vi "File Manager.vi"(0 "File Name":string, 1 "File Choice":T3, 3 "Existing Time":dbl, 4 "Voltage":waveform(dbl)[](array[waveform]), 5 "error in":errorcluster, 6 "Enum":T2=enum."Close File", 7 "Record Time (s)":dbl=10.0, 12 "Volt Channel":T1={"Index"=[], "Chl Name"=[], "Scale"=[], "Offset"=[], "Sample Rate"=100, "Device Name"="", "Channel"=""}, 13 "Use Record Time":bool) -> (14 "File Path":path, 15 "timeout":i32, 16 "ET out":dbl, 17 "Recording":bool, 18 "dt Out":dbl, 19 "error out":errorcluster)   [LabVIEW 2021]
doc: "This vi has four functions:\nCreate File - Create a new TDMS or CSV file depending on user choice. If user filled in file name, use that file name with time infomation. If user didn't filled in file name, use \"Experiment Result \"+time information.\nConfig Data - Save Channel Number, Channel Name, Scale and Offset into file.\nVolt Data - Create Time array and merge with Voltage Data, then save them into file. \nClost File - Close file and reset all parameters."
uses:
  Control/File Choice Enum.ctl
  Control/File Manager Enum.ctl
  Control/Volt Chl.ctl
  File Abstract Class/File Abstract.lvclass
  TDMS File Class/TDMS File.lvclass
  CSV File Class/CSV File.lvclass
  Control/File Information Cluster.ctl
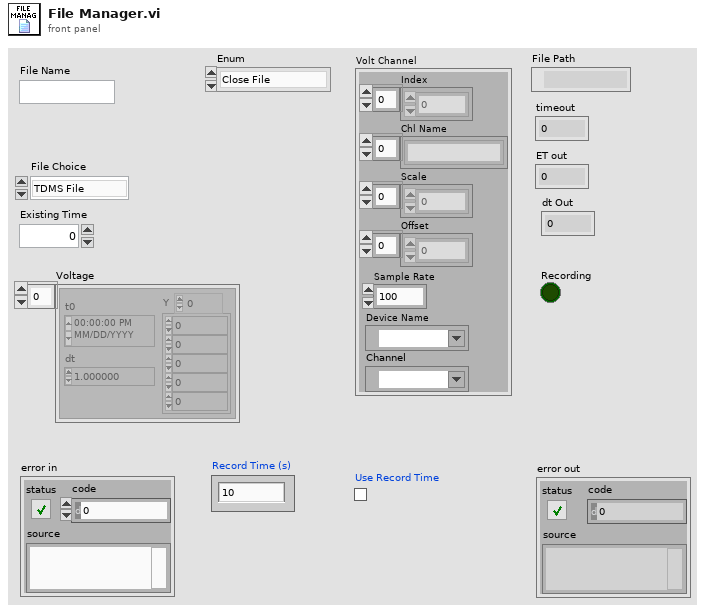
[diagram p1: front panel]
types:
  T1 = typedef "Volt Chl.ctl" = cluster{"Index":i32[], "Chl Name":string[], "Scale":dbl[], "Offset":dbl[], "Sample Rate":i32, "Device Name":tag, "Channel":tag}
  T2 = typedef "File Manager Enum.ctl" = enum16{"Create File", "Config Data", "Volt Data", "Set Time", "Close File"}
  T3 = typedef "File Choice Enum.ctl" = enum16{"TDMS File", "CSV File"}
  T4 = typedef "File Information Cluster.ctl" = cluster{"File Refnum":variant, "Chl Name":string[]}
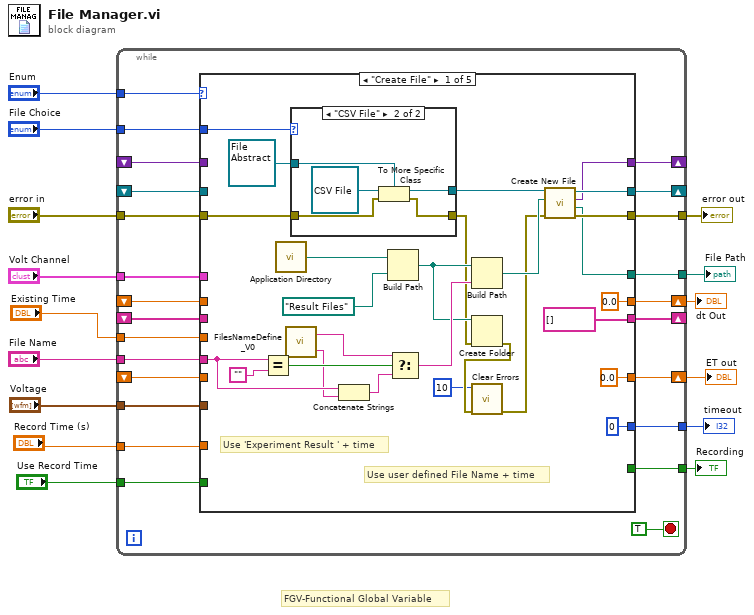
[diagram p0: block diagram]
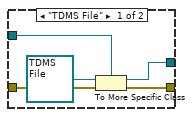
[diagram p2: hidden frame]
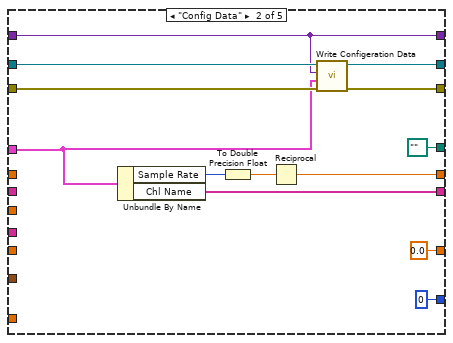
[diagram p3: hidden frame]
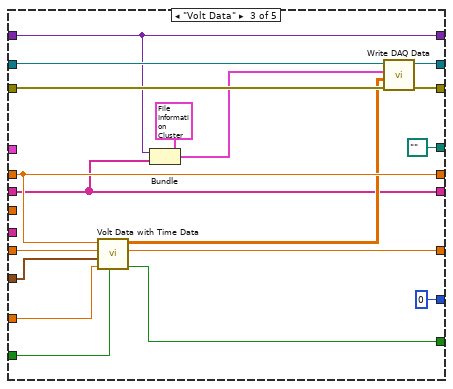
[diagram p4: hidden frame]
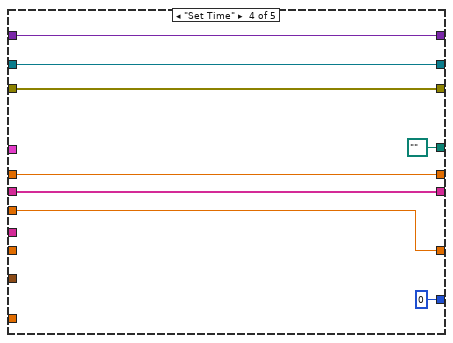
[diagram p5: hidden frame]
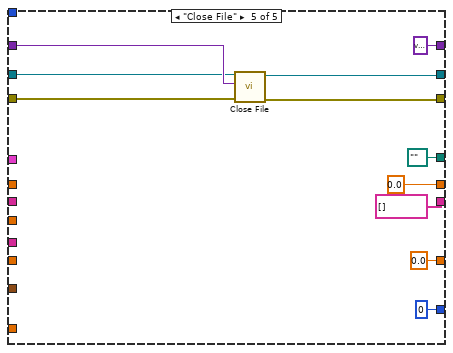
[diagram p6: hidden frame]
diagram:
  # "FGV-Functional Global Variable"
  n1 = while {
    tunnel: "File Name" -> [w39]
    tunnel: "File Choice" -> [w38]
    tunnel: [w35] -> w13
    shift-right: [w36] -> _
    shift-left: _ -> [w32]
    tunnel: "error in" -> [w34]
    tunnel: "Enum" -> [w33]
    tunnel: "Volt Channel" -> [w31]
    shift-right: [w30] -> _
    shift-left: _ -> [w29]
    tunnel: [w28] -> w9
    shift-right: [w27] -> w1
    shift-left: _ -> [w26]
    shift-right: [w25] -> _
    shift-left: _ -> [w24]
    shift-right: [w23] -> w2
    shift-left: _ -> [w22]
    tunnel: "Voltage" -> [w21]
    tunnel: "Record Time (s)" -> [w20]
    tunnel: [w19] -> w6
    tunnel: "Use Record Time" -> [w18]
    tunnel: [w17] -> w4
    tunnel: "Existing Time" -> [w16]
    stop <- TRUE stop-if-true
    n2 = case shown="\"Create File\"" w33 {
      tunnel: w39 -> [w48 _ _ _ _]
      tunnel: w38 -> [w64 _ _ _ _]
      tunnel: [w63 w88 w104 w110 w122] -> w36
      tunnel: [w62 w87 w105 w109 w123] -> w35
      tunnel: w34 -> [w61 w86 w106 w109 w124]
      tunnel: w32 -> [_ w89 w107 w110 w125]
      tunnel: w31 -> [_ w83 _ _ _]
      tunnel: [w60 w85 w101 w115 variant ("File Refnum")] -> w30
      tunnel: w29 -> [_ w85 w101 w115 w126]
      tunnel: [w54 path "" ("appended path") path "" ("appended path") path "" ("appended path") path "" ("appended path")] -> w28
      tunnel: [0.0 w80 w99 w113 0.0] -> w27
      tunnel: w26 -> [_ _ w99 w113 _]
      tunnel: [string[] [] ("Chl Name") w79 w96 w112 string[] [] ("Chl Name")] -> w25
      tunnel: w24 -> [_ _ w96 w112 _]
      tunnel: [0.0 0.0 w94 w108 0.0 ("t_start out")] -> w23
      tunnel: w22 -> [_ _ w95 _ _]
      tunnel: w21 -> [_ _ w98 _ _]
      tunnel: w20 -> [_ _ w93 _ _]
      tunnel: [0 ("timeout") 0 ("timeout") 0 ("timeout") 0 ("timeout") 0 ("timeout")] -> w19
      tunnel: w18 -> [_ _ w92 _ _]
      tunnel: [_ _ w91 _ _] -> w17
      tunnel: w16 -> [_ _ _ w108 _]
      frame "Create File" {
        # "Use 'Experiment Result ' + time"
        # "Use user defined File Name + time"
        n3 = Equal?(x=w48, y="") -> (x = y?=w57:bool)
        n4 = call <vilib>:"Application Directory.vi"() -> ("Application Directory"=w45:path)
        n5 = call "FilesNameDefine_V0.vi"() -> ("date/time string"=w47:string, "Result File Name"=w49:string)  [unwired: 2 in]
        n6 = case shown="\"CSV File\"" w64 {
          tunnel: refnum<class "File Abstract.lvclass"> refnum ("File Manager.lvclass") -> [w70 w76]
          tunnel: [w68 w74] -> w43
          tunnel: [w69 w73] -> w66
          tunnel: w61 -> [w67 w72]
          frame "TDMS File" {
            n7 = To More Specific Class(target class=w70, reference=refnum<class "TDMS File.lvclass"> refnum ("TDMS File.lvclass"), error in=w67) -> (specific class reference=w69:refnum<class "File Abstract.lvclass">, error out=w68:errorcluster)
          }
          frame "CSV File" {
            n8 = To More Specific Class(target class=w76, reference=refnum<class "CSV File.lvclass"> refnum ("CSV File.lvclass"), error in=w72) -> (specific class reference=w73:refnum<class "File Abstract.lvclass">, error out=w74:errorcluster)
          }
        }
        n9 = Concatenate Strings(w48, w47) -> (w46:string)
        n10 = Build Path(base path=w45, name or relative path=path "Result Files") -> (appended path=w44:path)
        n11 = Select(t=w49, s=w57, f=w46) -> (s? t:f=w56:string)
        n12 = Build Path(base path=w44, name or relative path=w56) -> (appended path=w55:path)
        n13 = Create Folder(path (use dialog)=w44, error in=w43) -> (error out=w42:errorcluster)  [unwired: 1 in, 2 out]
        n14 = call <vilib>:"Clear Errors.vi"("error in (no error)"=w42, "specific error code to clear (0: all)"=10) -> ("error out"=w40:errorcluster)  [unwired: 4 in, 1 out]
        n15 = call-dynamic "Create New File.vi"("error in (no error)"=w40, "Path"=w55, "File Manager in"=w66) -> ("error out"=w62:errorcluster, "Path out"=w54:path, "File Refnum"=w60:variant, "File Manager out"=w63:refnum<class "File Abstract.lvclass">)  [unwired: 5 in]
      }
      frame "Config Data" {
        n16 = Unbundle By Name(w83) -> ("Sample Rate"=w82:i32, "Chl Name"=w79:string[])
        n17 = To Double Precision Float(number=w82) -> (double precision float=w81:dbl)
        n18 = Reciprocal(x=w81) -> (1/x=w80:dbl)
        n19 = call-dynamic "Write Configeration Data.vi"("error in (no error)"=w86, "Volt Channel"=w83, "File Refnum"=w85, "File Manager in"=w89) -> ("error out"=w87:errorcluster, "File Manager out"=w88:refnum<class "File Abstract.lvclass">)  [unwired: 6 in]
      }
      frame "Volt Data" {
        n20 = call "Volt Data with Time Data.vi"("Use Record Time"=w92, "Record Time (s)"=w93, "Voltage"=w98, "t_start in"=w95, "dt"=w99) -> ("Recording"=w91:bool, "t_start out"=w94:dbl, "Data with Time"=w97:dbl[][])  [unwired: 3 in, 1 out]
        n21 = Bundle(cluster=T4 {"File Refnum"=variant, "Chl Name"=[]} ("File Infor"), "File Refnum"=w101, "Chl Name"=w96) -> (w102:T4)
        n22 = call-dynamic "Write DAQ Data.vi"("error in (no error)"=w106, "Voltage with Time"=w97, "File Infor"=w102, "File Manager in"=w107) -> ("error out"=w105:errorcluster, "File Manager out"=w104:refnum<class "File Abstract.lvclass">)  [unwired: 6 in]
      }
      frame "Set Time" {
      }
      frame "Close File" {
        n23 = call-dynamic "Close File.vi"("error in (no error)"=w124, "File Refnum"=w126, "File Manager in"=w125) -> ("error out"=w123:errorcluster, "File Manager out"=w122:refnum<class "File Abstract.lvclass">)  [unwired: 7 in]
      }
    }
  }
  "error out" <- w13
  "File Path" <- w9
  "timeout" <- w6
  "Recording" <- w4
  "ET out" <- w2
  "dt Out" <- w1
